vi "New XWPF Writer.vi"(8 "error in (no error)":errorcluster) -> (0 "error out":errorcluster, 3 "xwpfWriter out":refnum<class "xwpfWriter.lvclass">)   [LabVIEW 2017, in "LabVIEW NPOI.lvlib" / "xwpfWriter.lvclass"]
doc: "Creates an XWPFDocument as an input document. \nCreates an XWPFExtractor object using the input document."
uses:
  xwpfWriter.lvclass
  C:/Users/Neo/Desktop/Dev_Tools_BR/LabVIEW_NPOI/lib/NPOI 2.1.1/NPOI.OOXML.dll
  lib/NPOI 2.1.1/NPOI.OOXML.dll
  xwpfWriter.lvclass/xwpfWriter.ctl
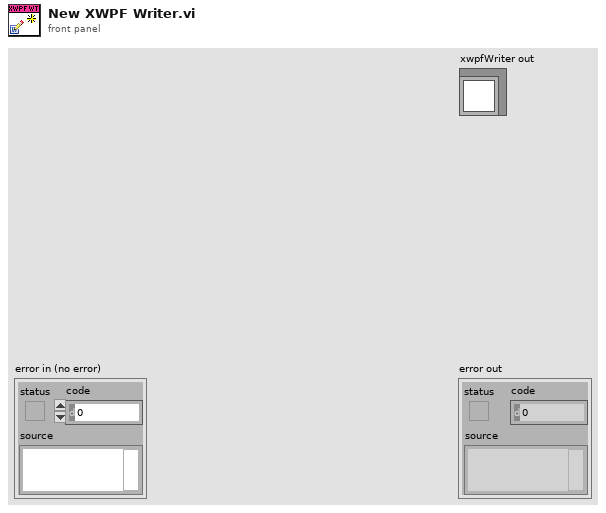
[diagram p1: front panel]
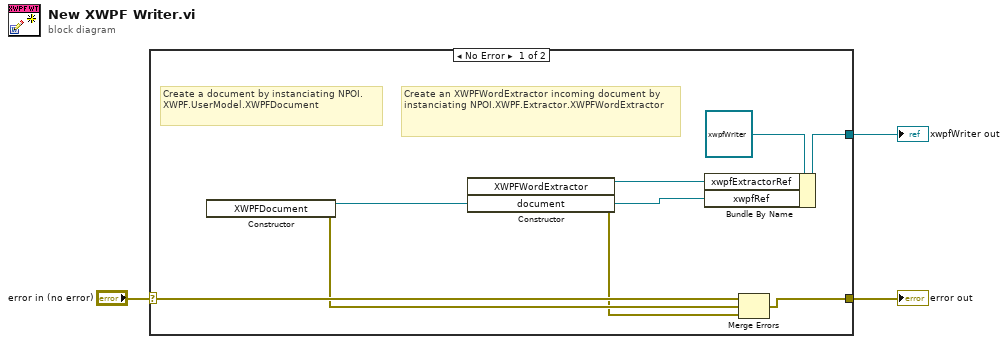
[diagram p0: block diagram]
diagram:
  n1 = case shown="No Error" "error in (no error)" {
    selector: "error in (no error)" -> [w11 w12]
    tunnel: [w10 w12] -> w2
    tunnel: [w8 _] -> w1
    frame No Error {
      # "Create an XWPFWordExtractor incoming document by instanciating NPOI.XWPF.Extractor.XWPFWordExtractor"
      # "Create a document by instanciating NPOI.XWPF.UserModel.XWPFDocument"
      n2 = constructor class="XWPFDocument"() -> (reference out=w4:refnum<k24>, error out=w6:errorcluster)  [unwired: 3 in, 1 out]
      n3 = constructor class="XWPFWordExtractor"("document"=w4) -> (reference out=w7:refnum<k24>, error out=w5:errorcluster)  [unwired: 3 in, 2 out]
      n4 = Bundle By Name(cluster=refnum<class "xwpfWriter.lvclass"> refnum ("xwpfWriter in"), "xwpfExtractorRef"=w7, "xwpfRef"=w4) -> (w8:refnum<class "xwpfWriter.lvclass">)
      n5 = Merge Errors(w11, w6, w5) -> (w10:errorcluster)
    }
    frame Error {
    }
  }
  "error out" <- w2
  "xwpfWriter out" <- w1
